vi "Write state.vi"(8 "error in (no error)":errorcluster, 10 "MountTrackStates":T1, 11 "MccAzElTrack in":refnum<class "MccAzElTrack.lvclass">) -> (0 "error out":errorcluster, 3 "MccAzElTrack out":refnum<class "MccAzElTrack.lvclass">)   [LabVIEW 2022 SP3, in "TCSDataDefinitions.lvlib" / "TCSMountControlCommand.lvlib" / "CommandsForAzElAxes.lvlib" / "MccAzElTrack.lvclass"]
uses:
  MccAzElTrack.lvclass
  Enumerations/MountTrackStates.ctl
  MccAzElTrack.lvclass/MccAzElTrack.ctl
  TCSMountControlCommand.lvlib
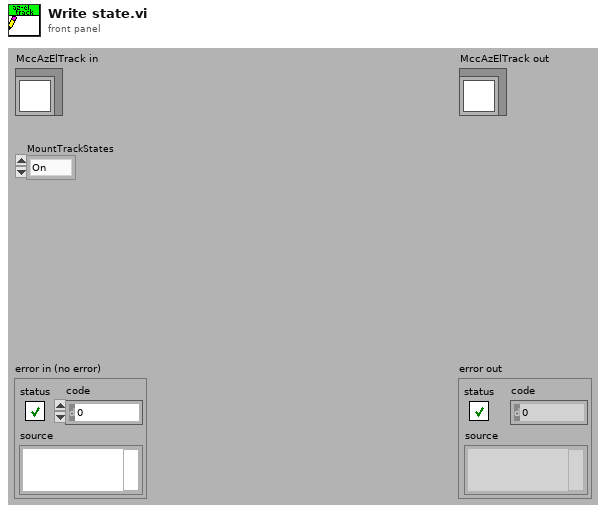
[diagram p1: front panel]
types:
  T1 = typedef "TCSDataDefinitions.lvlib/TCSMountControlCommand.lvlib/MountTrackStates.ctl" = enum16{"On", "Off"}
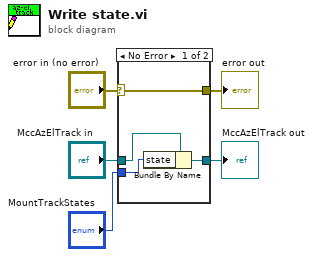
[diagram p0: block diagram]
diagram:
  n1 = case shown="No Error" "error in (no error)" {
    selector: "error in (no error)" -> [w9 w10]
    tunnel: [w9 w10] -> w4
    tunnel: [w7 w11] -> w2
    tunnel: "MccAzElTrack in" -> [w8 w11]
    tunnel: "MountTrackStates" -> [w6 _]
    frame No Error {
      n2 = Bundle By Name(cluster=w8, "state"=w6) -> (w7:refnum<class "MccAzElTrack.lvclass">)
    }
    frame Error {
    }
  }
  "error out" <- w4
  "MccAzElTrack out" <- w2
